vi "Create Transfers.vi"(5 "Group String Buffer":refnum<class "Buffer.lvclass">, 7 "Group Intermediate Buffer":refnum<class "DBL Pointer.lvclass">, 8 "error in (no error)":errorcluster, 10 "Transfer Configurations":T1[](array[typedef]) {"channel configurations"."buffer offset" format="%d bytes"}, 11 "Framework in":refnum<class "Framework.lvclass">) -> (0 "error out":errorcluster, 2 "Transfers":refnum<class "Transfer.lvclass">[](array[class]), 3 "Framework out":refnum<class "Framework.lvclass">)   [LabVIEW 2017, in "DSF Core.lvlib" / "Framework.lvclass"]
uses:
  Framework.lvclass
  Transfer/Transfer.lvclass
  Configuration/Public/Controls/DSF Engine Transfer Configuration.ctl
  Configuration/Public/Controls/DSF Byte Order.ctl
  Configuration/Public/Controls/DSF Engine Channel Configuration.ctl
  Configuration/Public/Controls/DSF Data Type.ctl
  Configuration/Public/Controls/DSF Settings Info.ctl
  Buffer/Buffer.lvclass
  C:/Program Files (x86)/National Instruments/LabVIEW 2017/vi.lib/NI/Memory Manager/Classes/Pointer/Pointer.lvclass
  Pointer/DBL Pointer.lvclass
  Framework.lvclass/Framework.ctl
  Cache/Cache.lvclass/Cache.ctl
  <vilib>/NI/Memory Manager/Classes/Pointer/Pointer.lvclass/Pointer.ctl
  VIs/Sizeof.vi
  <vilib>/NI/Memory Manager/Classes/Pointer/Protected/Parameter Checking/Check Subset.vi
  <vilib>/NI/Memory Manager/Classes/Pointer/API/Accessors/Get Address.vi
  <vilib>/NI/Memory Manager/Classes/Pointer/API/Encapsulate External Pointer.vi
  <vilib>/NI/Memory Manager/Classes/Pointer/Protected/Parameter Checking/Check Null Pointer.vi
  <vilib>/NI/Memory Manager/Classes/Pointer/Protected/Errors.vi
  <vilib>/NI/Memory Manager/Classes/Pointer/Protected/Error VIs/Out of Bounds.vi
  <vilib>/NI/Memory Manager/Classes/Pointer/API/Accessors/Get Size.vi
  <vilib>/NI/Memory Manager/Classes/Pointer/API/Accessors/Set Size.vi
  <vilib>/NI/Memory Manager/Classes/Pointer/API/Accessors/Set Address.vi
  <vilib>/NI/Memory Manager/Classes/Pointer/Private/Set Internal.vi
  <vilib>/NI/Memory Manager/Classes/Pointer/Protected/Error VIs/Null Pointer.vi
  <vilib>/NI/Memory Manager/VIs/Write String into Source.vi
  <vilib>/NI/Memory Manager/Classes/Pointer/Protected/Error Building/Write Pointer Size.vi
  <vilib>/NI/Memory Manager/Classes/Pointer/Protected/Error Building/Create Error.vi
  <vilib>/NI/Memory Manager/VIs/Write Number into Source.vi
  <vilib>/NI/Memory Manager/VIs/VIs for Poly/Write U64 into Source.vi
  <vilib>/NI/Memory Manager/Constants/Constants.vi
  <vilib>/NI/Memory Manager/Constants/Library Name.vi
  <vilib>/NI/Memory Manager/Classes/Pointer/Protected/Error Building/Get Error Info.vi
  <vilib>/NI/Memory Manager/VIs/Create Error Cluster.vi
  <vilib>/NI/Memory Manager/VIs/VIs for Poly/Create Error Cluster (256B).vi
  <vilib>/NI/Memory Manager/VIs/Set Error Status.vi
  <vilib>/NI/Memory Manager/VIs/Set Error Code.vi
  <vilib>/NI/Memory Manager/VIs/Set Error Source.vi
  DSF Core.lvlib
  Cache/Cache.lvclass
  <vilib>/NI/Memory Manager/Classes/Pointer/Pointer.lvclass
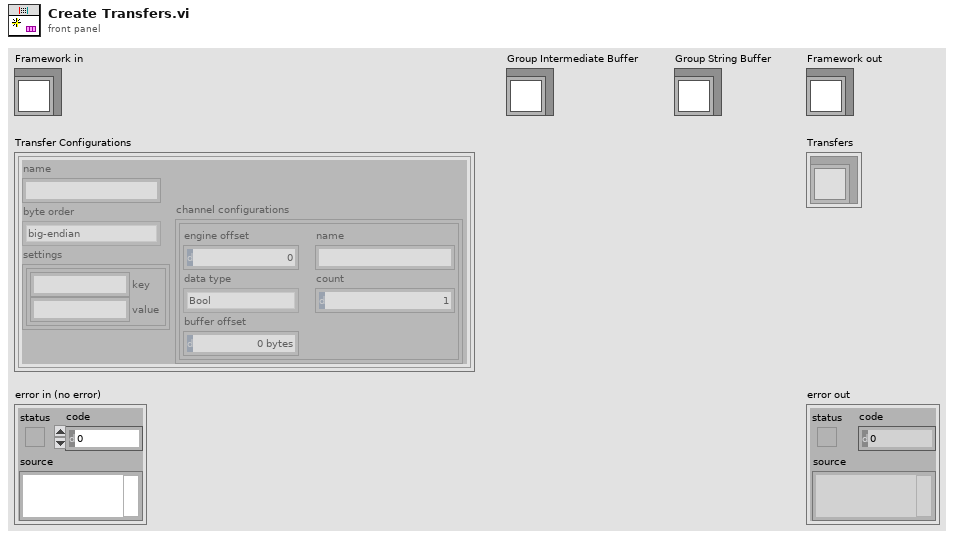
[diagram p1: front panel]
types:
  T1 = typedef "DSF Core.lvlib/DSF Engine Transfer Configuration.ctl" = cluster{"name":string, "byte order":T2, "channel configurations":T3[], "settings":T5}
  T2 = typedef "DSF Core.lvlib/DSF Byte Order.ctl" = enum8{"big-endian", "little-endian"}
  T3 = typedef "DSF Core.lvlib/DSF Engine Channel Configuration.ctl" = cluster{"engine offset":u64, "name":string, "data type":T4, "count":u64, "buffer offset":u64}
  T4 = typedef "DSF Core.lvlib/DSF Data Type.ctl" = enum8{"Bool", "SGL", "DBL", "I8", "I16", "I32", "I64", "U8", "U16", "U32", "U64"}
  T5 = typedef "DSF Core.lvlib/DSF Settings Info.ctl" = cluster{"key":string, "value":string}[]
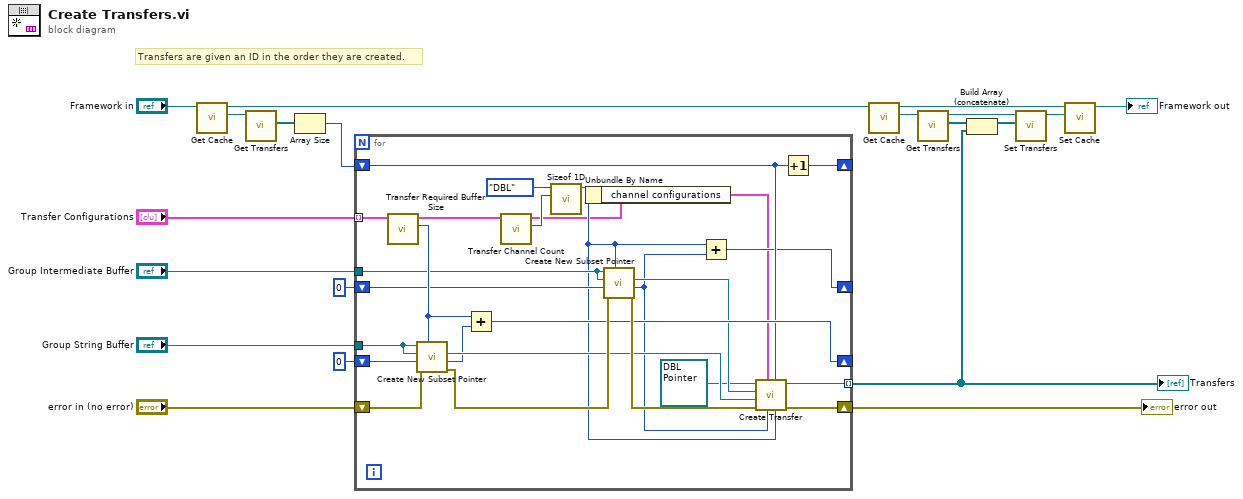
[diagram p0: block diagram]
diagram:
  # "Transfers are given an ID in the order they are created."
  n1 = call "Get Cache.vi"("Framework in"="Framework in") -> ("Cache"=w14:refnum<class "Cache.lvclass">, "Framework out"=w12:refnum<class "Framework.lvclass">)  [unwired: 9 in]
  n2 = call "Get Transfers.vi"("Cache in"=w14) -> ("Transfers"=w16:refnum<class "Transfer.lvclass">[])  [unwired: 9 in, 1 out]
  n3 = Array Size(array=w16) -> (size(s)=w17:i32)
  n4 = for {
    shift-right: [w44] -> w20
    shift-left: "error in (no error)" -> [w35]
    tunnel: [w43] -> w10 mode=indexing
    tunnel: "Transfer Configurations" -> [w41] mode=indexing
    tunnel: "Group Intermediate Buffer" -> [w28]
    shift-right: [w29] -> _
    shift-left: u64 0 -> [w26]
    tunnel: "Group String Buffer" -> [w33]
    shift-right: [w36] -> _
    shift-left: u64 0 -> [w39]
    shift-right: [w31] -> _
    shift-left: w17 -> [w30]
    n5 = call "Transfer Required Buffer Size.vi"("Transfer Configuration in"=w41) -> ("required buffer size"=w38:u64, "Transfer Configuration out"=w40:T1)  [unwired: 8 in, 1 out]
    n6 = call <vilib>:"Create New Subset Pointer.vi"("length (-1: rest)"=w38, "error in (no error)"=w35, "offset (0)"=w39, "subset Pointer type"=w33, "base Pointer in"=w33) -> ("error out"=w46:errorcluster, "offset out"=w34:u64, "subset Pointer"=w37:refnum<class "Buffer.lvclass">)  [unwired: 3 in, 1 out]
    n7 = Add(x=w38, y=w34) -> (x+y=w36:u64)
    n8 = call "Transfer Channel Count.vi"("Transfer Configuration in"=w40) -> ("total channel count"=w32:u64, "Transfer Configuration out"=w22:T1)  [unwired: 8 in, 1 out]
    n9 = call "Sizeof 1D.vi"("count"=w32, "data type"=DSF_Data_Type."DBL") -> ("size in bytes"=w23:u64)  [unwired: 9 in]
    n10 = Unbundle By Name(w22) -> ("channel configurations"=w21:T3[])
    n11 = call <vilib>:"Create New Subset Pointer.vi"("length (-1: rest)"=w23, "error in (no error)"=w46, "offset (0)"=w26, "subset Pointer type"=w28, "base Pointer in"=w28) -> ("error out"=w45:errorcluster, "offset out"=w24:u64, "subset Pointer"=w27:refnum<class "DBL Pointer.lvclass">)  [unwired: 3 in, 1 out]
    n12 = Add(x=w23, y=w24) -> (x+y=w29:u64)
    n13 = call "Create Transfer.vi"("size"=w23, "id"=w30, "group offset"=w24, "channel blocks"=w21, "error in (no error)"=w45, "String Buffer"=w37, "Intermediate Buffer"=w27, "Inline Buffer"=refnum<class "DBL Pointer.lvclass"> refnum) -> ("error out"=w44:errorcluster, "Transfer out"=w43:refnum<class "Transfer.lvclass">)  [unwired: 2 in]
    n14 = Increment(x=w30) -> (x+1=w31:i32)
  }
  "error out" <- w20
  "Transfers" <- w10
  n15 = call "Get Cache.vi"("Framework in"=w12) -> ("Cache"=w13:refnum<class "Cache.lvclass">, "Framework out"=w9:refnum<class "Framework.lvclass">)  [unwired: 9 in]
  n16 = call "Get Transfers.vi"("Cache in"=w13) -> ("Transfers"=w11:refnum<class "Transfer.lvclass">[], "Cache out"=w5:refnum<class "Cache.lvclass">)  [unwired: 9 in]
  n17 = Build Array (concatenate)(w11, w10) -> (w8:refnum<class "Transfer.lvclass">[])
  n18 = call "Set Transfers.vi"("Transfers"=w8, "Cache in"=w5) -> ("Cache out"=w7:refnum<class "Cache.lvclass">)  [unwired: 9 in]
  n19 = call "Set Cache.vi"("Cache"=w7, "Framework in"=w9) -> ("Framework out"=→"Framework out":refnum<class "Framework.lvclass">)  [unwired: 9 in]
